vi "Immediate_Pullup_Winch.vi"(2 "Percent Output":dbl) -> (10 "Command Info Out":T1)   [LabVIEW 2019]
doc: "This template is useful for immediate subsystem actions that do not need deadband filtering\n\nBe sure to right-click and select New from Template and save with a new command name."
uses:
  <vilib>/Rock Robotics/WPI/Framework/Command Status Info.ctl
  <vilib>/Rock Robotics/WPI/Framework/Completion Status.ctl
  <vilib>/Rock Robotics/WPI/Framework/Completion Notifier.ctl
  Implementation/Winches Setpoints.ctl
  Implementation/Winches Operations.ctl
panel:
  in  "Command Info In":T1
  in  "Description":string
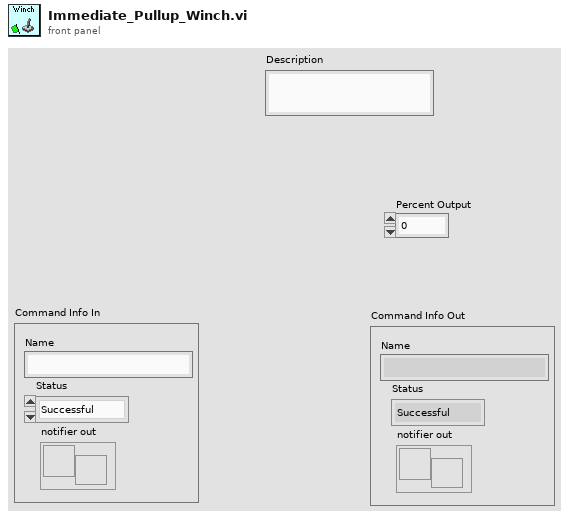
[diagram p1: front panel]
types:
  T1 = typedef "Command Status Info.ctl" = cluster{"Name":string, "Status":T2, "notifier out":T3}
  T2 = typedef "Completion Status.ctl" = enum16{"Successful", "Aborted", "Incomplete"}
  T3 = typedef "Completion Notifier.ctl" = refnum<notifier>
  T4 = typedef "Winches Setpoints.ctl" = cluster{"Operation":T5, "Percent Power":dbl}
  T5 = typedef "Winches Operations.ctl" = enum16{"Reserve", "Read Current", "Actuate Lift", "Actuate Telescope"}
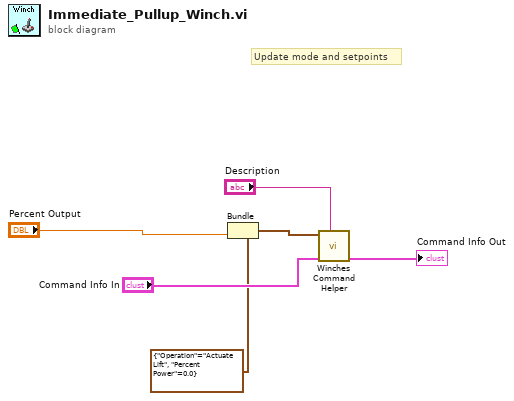
[diagram p0: block diagram]
diagram:
  # "Update mode and setpoints"
  n1 = Bundle(cluster=T4 {"Operation"=enum."Actuate Lift", "Percent Power"=0.0} ("SubSystem Data"), "Percent Power"="Percent Output") -> (w2:T4)  [unwired: 1 in]
  n2 = call "Winches Command Helper.vi"("Description"="Description", "Command Info In"="Command Info In", "SubSystem Data"=w2) -> ("Command Info Out"=→"Command Info Out":T1)  [unwired: 6 in, 2 out]
